vi "Rx Packet Page.vi"(8 "error in (no error)":errorcluster, 11 "Node Ptr":T2 format="%.0x") -> (0 "error out":errorcluster)   [LabVIEW 2023, in "UDP-Custom-Device System Explorer.lvlib"]
uses:
  UDP-Custom-Device System Explorer.lvlib
  Shared/Types/Shared - New Data Options.ctl
  <vilib>/NI VeriStand/Custom Device API/Custom Device Item Ref.ctl
  Types/Page References/Refs - Rx Packets Page.ctl
  Shared/Types/Shared - Channel Data Type.ctl
  <vilib>/NI VeriStand/Custom Device API/Custom Device API.lvlib
  Property Accessors/Shared Packet Accessors.lvlib
  <vilib>/NI VeriStand/Custom Device Tools/Custom Device Utility Library/Custom Device Utility Library.lvlib
  Property Accessors/Rx Channel Accessors.lvlib
  Property Accessors/Rx Packet Accessors.lvlib
  Property Accessors/Rx Channel Section Accessors.lvlib
  Shared/UDP-Custom-Device Shared.lvlib
panel:
  in  "Config Threading":bool
  in  "Debug Mode":bool caption="Auto-Assign Local NIC"
  in  "New Data Options":T1
  in  "Multicast IP Address":string
  in  "Multicast?":bool caption="Auto-Assign Local NIC"
  in  "Read Timeout (ms)":i32
  in  "Channel Config Export":bool
  in  "Configure Header":bool
  in  "Endianness":u16(ring) items=["big-endian"=0, "little-endian"=2]
  in  "General Header 3":cluster{"Section Name":string}={"Section Name"="Network Settings"}
  out "Packet ID":i32
  in  "Auto-Assign Local NIC":bool
  in  "Port":u16
  in  "IP Address of Local NIC":string
  in  "Description":string
  in  "Name":string
  in  "General Header 2":cluster{"Section Name":string}={"Section Name"="Configured Channels"}
  in  "Rx Channels":i32[](listbox)
  in  "SHDocVw.IWebBrowser":refnum<k7>(container)
  in  "General Header":cluster{"Section Name":string}={"Section Name"="Packet Configuration"}
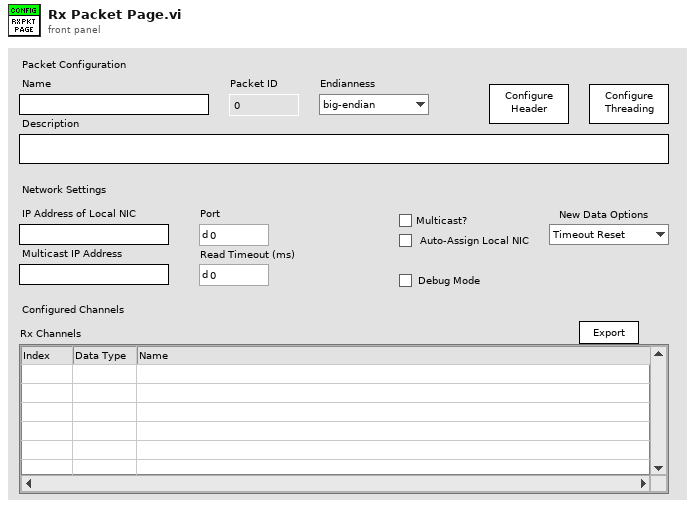
[diagram p1: front panel]
types:
  T1 = typedef "UDP-Custom-Device Shared.lvlib/Shared - New Data Options.ctl" = enum16{"Timeout Reset", "Counter"}
  T2 = typedef "Custom Device API.lvlib/Custom Device Item Ref.ctl" = u64
  T3 = typedef "UDP-Custom-Device System Explorer.lvlib/Refs - Rx Packets Page.ctl" = cluster{"Name":refnum<vi>, "Description":refnum<vi>, "Rx Packets":refnum<vi>, "Auto Assign Local NIC?":refnum<vi>, "IP Address of Local NIC":refnum<vi>, "Port":refnum<vi>, "Packet ID":refnum<vi>, "Channel Config Export":refnum<vi>, "Read Timeout (ms)":refnum<vi>, "Endianness":refnum<vi>, "Multicast IP Address":refnum<vi>, "Multicast?":refnum<vi>, "New Data Options":refnum<vi>, "Debug Mode":refnum<vi>}
  T4 = enum8{"Enabled", "Disabled", "Disabled and Grayed Out"}
  T5 = typedef "UDP-Custom-Device Shared.lvlib/Shared - Channel Data Type.ctl" = enum16{"Boolean", "Single", "Double", "I8", "I16", "I32", "I64", "U8", "U16", "U32", "U64"}
  T6 = typedef "Custom Device API.lvlib/Custom Device Commands.ctl" = enum16{"Default", "Item renamed", "Shutdown", "Dynamic button pressed"}
  T7 = typedef "UDP-Custom-Device System Explorer.lvlib/Thread Configuration.ctl" = cluster{"targetProcessor":i8, "targetPriority":i16, "Synchronization":T8, "loopPeriod":u32, "pclDecimation":u16, "threadManagement":T9}
  T8 = typedef "UDP-Custom-Device System Explorer.lvlib/Thread Sync Reference.ctl" = enum16{"PCL", "Async"}
  T9 = typedef "UDP-Custom-Device Shared.lvlib/Shared - Thread Management.ctl" = enum16{"Untimed (Default)", "Timed (High Priority)"}
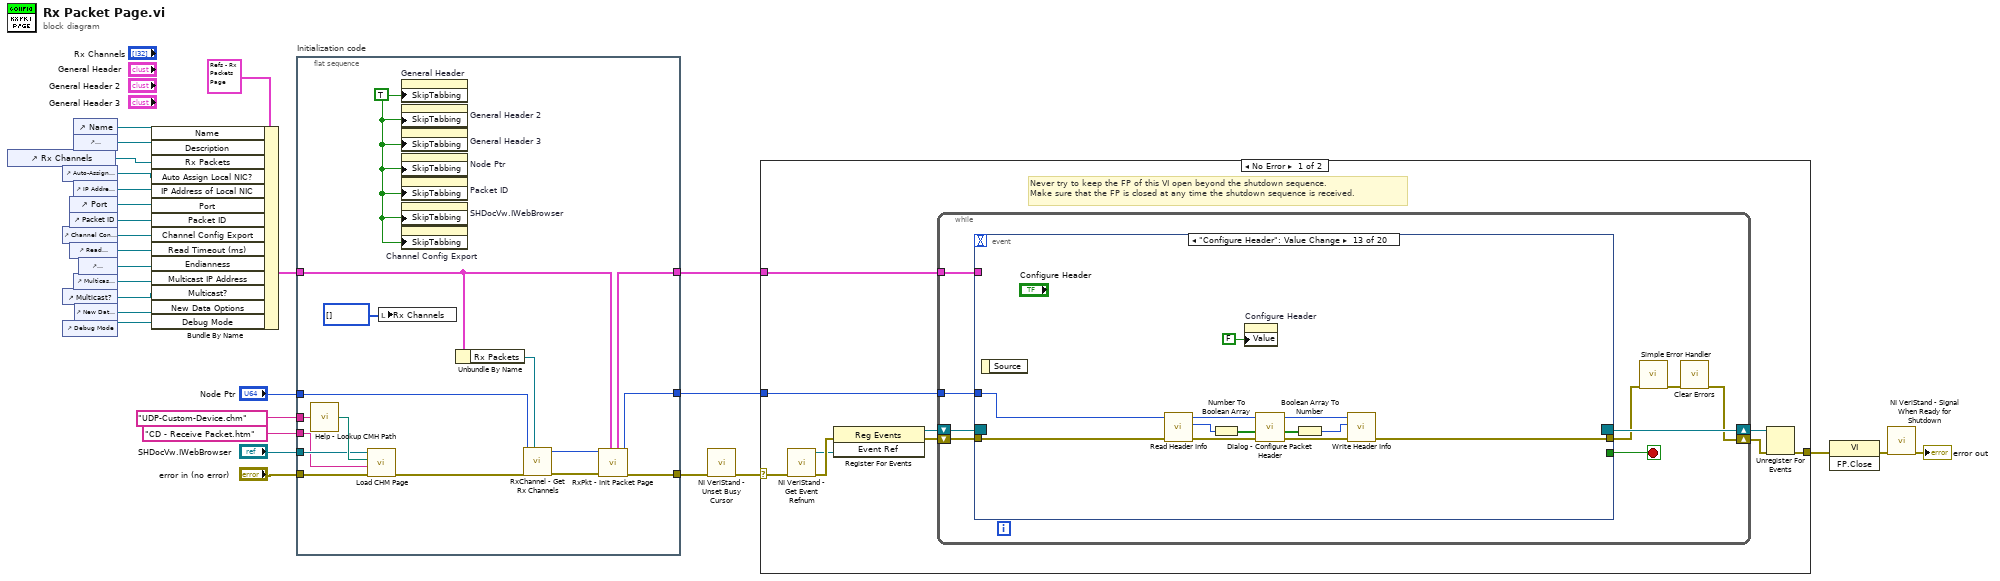
[diagram p0: block diagram]
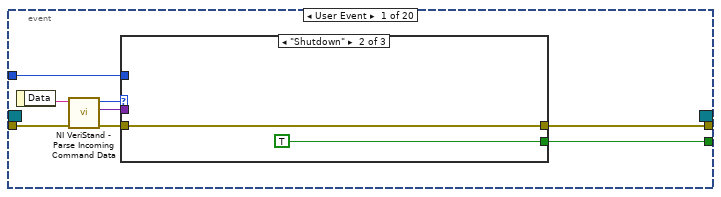
[diagram p2: hidden frame]
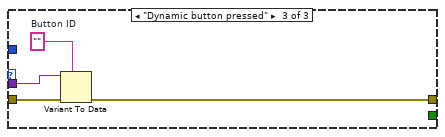
[diagram p4: hidden frame]
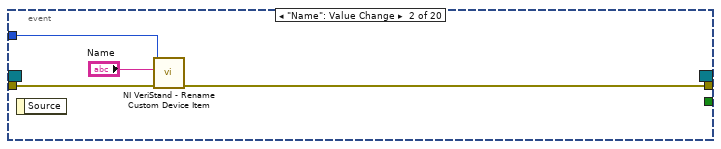
[diagram p5: hidden frame]
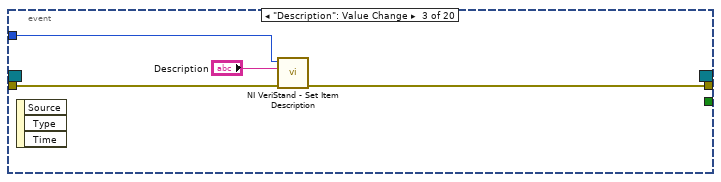
[diagram p6: hidden frame]
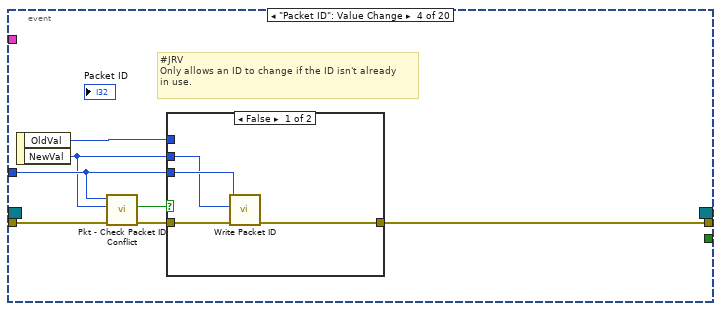
[diagram p7: hidden frame]
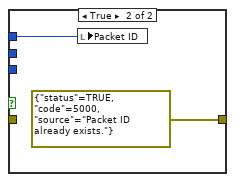
[diagram p8: hidden frame]
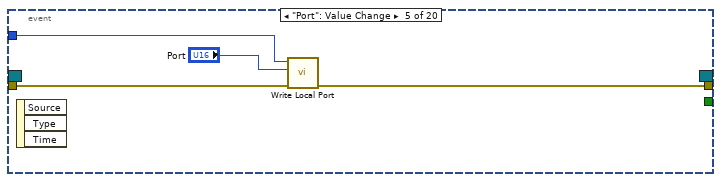
[diagram p9: hidden frame]
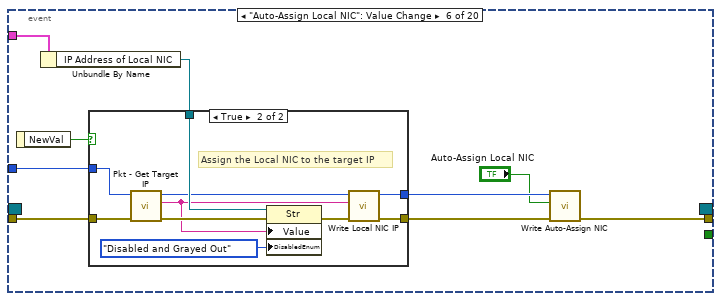
[diagram p10: hidden frame]
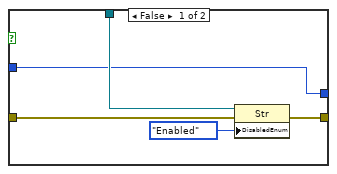
[diagram p11: hidden frame]
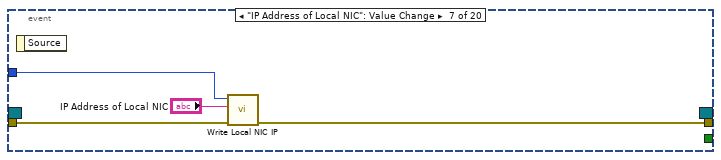
[diagram p12: hidden frame]
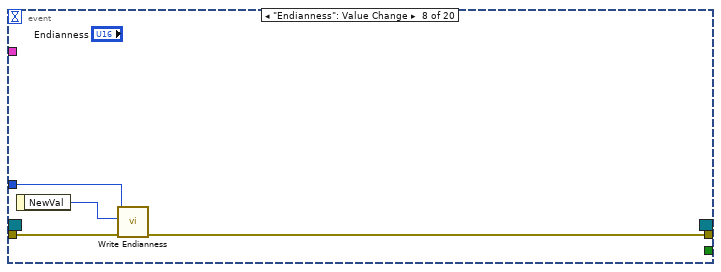
[diagram p13: hidden frame]
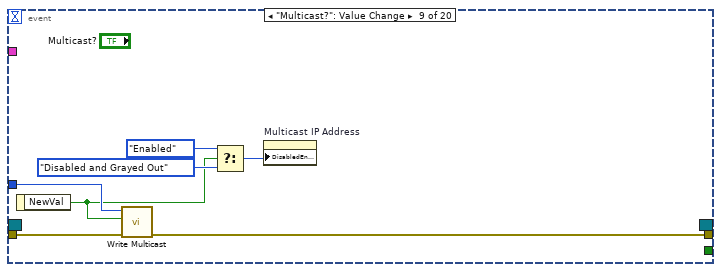
[diagram p14: hidden frame]
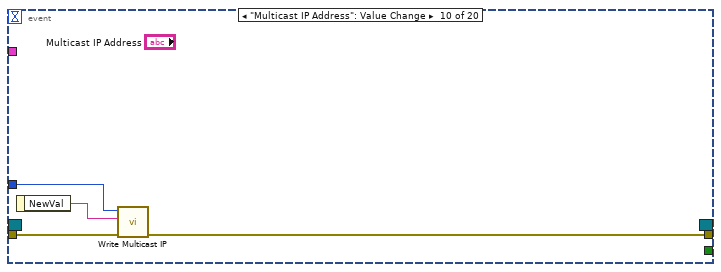
[diagram p15: hidden frame]
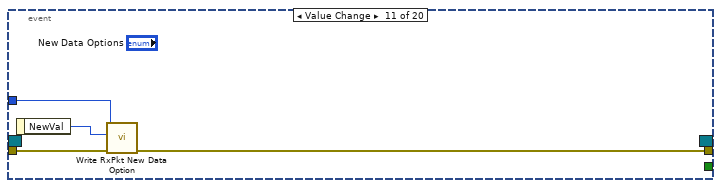
[diagram p16: hidden frame]
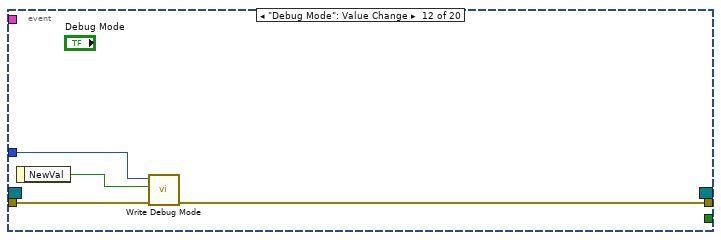
[diagram p17: hidden frame]
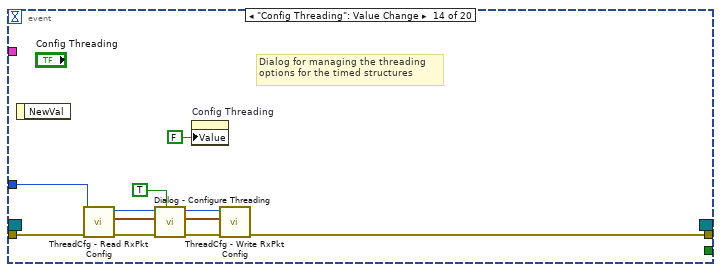
[diagram p18: hidden frame]
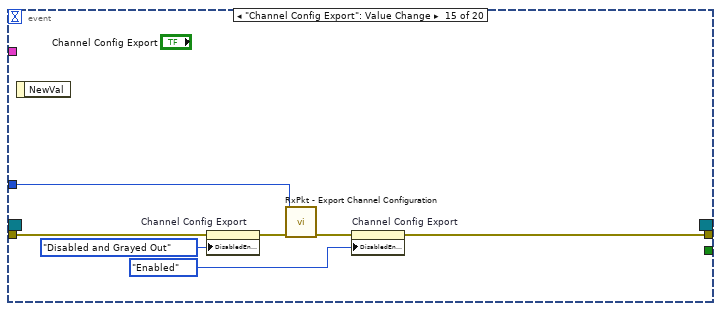
[diagram p19: hidden frame]
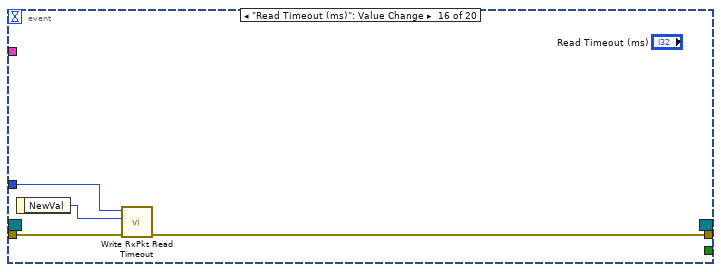
[diagram p20: hidden frame]
diagram:
  n1 = control-ref of="Rx Channels"() -> (w13:refnum<vi>)
  n2 = control-ref of="Auto-Assign Local NIC"() -> (w14:refnum<vi>)
  n3 = control-ref of="Channel Config Export"() -> (w7:refnum<vi>)
  n4 = control-ref of="Multicast?"() -> (w4:refnum<vi>)
  n5 = control-ref of="Debug Mode"() -> (w1:refnum<vi>)
  n6 = control-ref of="Port"() -> (w10:refnum<vi>)
  n7 = control-ref of="Packet ID"() -> (w12:refnum<vi>)
  n8 = control-ref of="Read Timeout (ms)"() -> (w6:refnum<vi>)
  n9 = control-ref of="Name"() -> (w16:refnum<vi>)
  n10 = control-ref of="Description"() -> (w15:refnum<vi>)
  n11 = control-ref of="IP Address of Local NIC"() -> (w11:refnum<vi>)
  n12 = control-ref of="Multicast IP Address"() -> (w3:refnum<vi>)
  n13 = control-ref of="New Data Options"() -> (w2:refnum<vi>)
  n14 = control-ref of="Endianness"() -> (w5:refnum<vi>)
  n15 = Bundle By Name(cluster=T3 {"Name"=refnum, "Description"=refnum, "Rx Packets"=refnum, "Auto Assign Local NIC?"=refnum, "IP Address of Local NIC"=refnum, "Port"=refnum, "Packet ID"=refnum, "Channel Config Export"=refnum, "Read Timeout (ms)"=refnum, "Endianness"=refnum, "Multicast IP Address"=refnum, "Multicast?"=refnum, "New Data Options"=refnum, "Debug Mode"=refnum} ("Rx Section Cluster"), "Name"=w16, "Description"=w15, "Rx Packets"=w13, "Auto Assign Local NIC?"=w14, "IP Address of Local NIC"=w11, "Port"=w10, "Packet ID"=w12, "Channel Config Export"=w7, "Read Timeout (ms)"=w6, "Endianness"=w5, "Multicast IP Address"=w3, "Multicast?"=w4, "New Data Options"=w2, "Debug Mode"=w1) -> (w9:T3)
  n16 = flat-sequence "Initialization code" {
    tunnel: "error in (no error)" -> [w38]
    tunnel: "Node Ptr" -> [w43]
    tunnel: [w31] -> w24
    tunnel: "SHDocVw.IWebBrowser" -> [w36]
    tunnel: "CD - Receive Packet.htm" ("CD_CHM_Section") -> [w35]
    tunnel: "UDP-Custom-Device.chm" ("CD_CHM_FileName") -> [w37]
    tunnel: w9 -> [w42]
    tunnel: [w41] -> w18
    tunnel: [w34] -> w8
    frame #0 {
      w29 = TRUE ("Skip When Tabbing")
      n17 = call "Help - Lookup CMH Path.vi"("Main CMH File"=w37) -> ("Compiled CMH Path"=w39:path)
      n18 = call <vilib>:"Load CHM Page.vi"("error in (no error)"=w38, "HTML File"=w35, "Compiled CHM Path"=w39, "Web Browser Reference"=w36) -> ("error out"=w30:errorcluster)  [unwired: 7 in]
      n19 = local write "Rx Channels"(i32[] [] ("Rx Channels")) -> ()
      n20 = property on="General Header" class="Clust (strict)"("SkipTabbing"=w29) -> ()  [unwired: 2 in, 2 out]
      n21 = property on="General Header 2" class="Clust (strict)"("SkipTabbing"=w29) -> ()  [unwired: 2 in, 2 out]
      n22 = property on="General Header 3" class="Clust (strict)"("SkipTabbing"=w29) -> ()  [unwired: 2 in, 2 out]
      n23 = property on="Node Ptr" class="DigNum (strict)"("SkipTabbing"=w29) -> ()  [unwired: 2 in, 2 out]
      n24 = property on="Packet ID" class="DigNum (strict)"("SkipTabbing"=w29) -> ()  [unwired: 2 in, 2 out]
      n25 = property on="SHDocVw.IWebBrowser" class="AXCont"("SkipTabbing"=w29) -> ()  [unwired: 2 in, 2 out]
      n26 = property on="Channel Config Export" class="Bool"("SkipTabbing"=w29) -> ()  [unwired: 2 in, 2 out]
      n27 = Unbundle By Name(w42) -> ("Rx Packets"=w44:refnum<vi>)
      n28 = call "RxChannel - Get Rx Channels.vi"("MCLB"=w44, "error in (no error)"=w30, "Node Ptr"=w43) -> ("error out"=w32:errorcluster, "Node Ptr out"=w40:T2)  [unwired: 6 in, 1 out]
      n29 = call "RxPkt - Init Packet Page.vi"("Rx Section Cluster In"=w42, "error in (no error)"=w32, "Node Ptr In"=w40) -> ("error out"=w31:errorcluster, "Node Ptr Out"=w34:T2, "Rx Section Cluster Out"=w41:T3)  [unwired: 6 in]
    }
  }
  n30 = call <vilib>:"NI VeriStand - Unset Busy Cursor.vi"("error in (no error)"=w24) -> ("error out"=w23:errorcluster)  [unwired: 10 out]
  n31 = case shown="No Error" w23 {
    selector: w23 -> [w46 w270]
    tunnel: [w51 w268] -> w28
    tunnel: w8 -> [w47 _]
    tunnel: w18 -> [w45 _]
    frame No Error {
      # "Never try to keep the FP of this VI open beyond the shutdown sequence.\nMake sure that the FP is closed at any time the shutdown sequence is received."
      n32 = call <vilib>:"NI VeriStand - Get Event Refnum.vi"("error in (no error)"=w46) -> ("error out"=w54:errorcluster, "Event Ref"=w50:refnum<user-event>)  [unwired: 9 out]
      n33 = register-events(error in=w54, w50) -> (reference out=w48:refnum<event-registration>, error out=w49:errorcluster)  [unwired: 1 in]
      n34 = while {
        tunnel: w47 -> [w59]
        shift-right: [w56] -> w52
        shift-left: w49 -> [w62]
        shift-right: [w63] -> w53
        shift-left: w48 -> [w61]
        tunnel: w45 -> [w55]
        stop <- w60 stop-if-true
        n35 = event shown="[12] \"Configure Header\": Value Change" {
          selector: w61 -> [_ _ _ _ _ _ _ _ _ _ _ _ _ _ _ _ _ _ _ _]
          dyn-events: [_ _ _ _ _ _ _ _ _ _ _ _ _ _ _ _ _ _ _ _] -> w63
          timeout: _ -> [_ _ _ _ _ _ _ _ _ _ _ _ _ _ _ _ _ _ _ _]
          tunnel: w62 -> [w71 w82 w86 w91 w102 w112 w131 w134 w141 w144 w148 w153 w163 w176 w183 w188 w190 w203 _ w225]
          tunnel: [w67 _ _ _ _ _ _ _ _ _ _ _ _ _ _ _ _ _ _ _] -> w60
          tunnel: [w66 w80 w83 w93 w101 w105 w130 w133 w140 w143 w147 w151 w157 w170 w180 w185 w189 w200 _ w226] -> w58
          tunnel: w59 -> [w65 w81 w85 w92 w103 w111 w128 w135 w142 w146 w150 w154 w164 w175 w184 w187 w191 w204 _ w224]
          tunnel: w55 -> [_ _ _ _ _ w108 _ _ _ _ _ _ _ _ _ _ _ _ _ _]
          event User Event {
            n36 = event-data() -> ("Data"=w70:string)  [unwired: 1 out]
            n37 = call <vilib>:"NI VeriStand - Parse Incoming Command Data.vi"("error in (no error)"=w71, "Incoming data"=w70) -> ("error out"=w69:errorcluster, "Outgoing data"=w64:variant, "Action"=w68:T6)  [unwired: 7 out]
            n38 = case shown="\"Shutdown\"" w68 {
              tunnel: w69 -> [w72 w73 w78]
              tunnel: [_ TRUE _] -> w67
              tunnel: [w72 w73 w75] -> w66
              tunnel: w65 -> [_ _ _]
              tunnel: w64 -> [_ _ w77]
              frame "Default", Default {
              }
              frame "Shutdown" {
              }
              frame "Dynamic button pressed" {
                w76 = ""  # Button ID
                n39 = Variant To Data(error in=w78, type=w76, Variant=w77) -> (error out=w75:errorcluster)  [unwired: 1 out]
              }
            }
          }
          event "Name": Value Change {
            n40 = event-data() -> ()  [unwired: 2 out]
            n41 = call <vilib>:"NI VeriStand - Rename Custom Device Item.vi"("error in (no error)"=w82, "New Name"="Name", "Item Ref in"=w81) -> ("error out"=w80:errorcluster)  [unwired: 6 in, 2 out]
          }
          event "Description": Value Change {
            n42 = event-data() -> ()  [unwired: 4 out]
            n43 = call <vilib>:"NI VeriStand - Set Item Description.vi"("error in (no error)"=w86, "Description"="Description", "Item Ref in"=w85) -> ("error out"=w83:errorcluster)  [unwired: 6 in, 2 out]
          }
          event "Packet ID": Value Change {
            # "#JRV\nOnly allows an ID to change if the ID isn't already\nin use."
            n44 = event-data() -> ("OldVal"=w87:i32, "NewVal"=w88:i32)  [unwired: 1 out]
            n45 = call "Pkt - Check Packet ID Conflict.vi"("error in (no error)"=w91, "New ID"=w88, "Packet Ref In"=w92) -> ("error out"=w90:errorcluster, "Conflicting ID?"=w89:bool)  [unwired: 7 in]
            n46 = case shown="False" w89 {
              tunnel: [w96 errorcluster {"status"=TRUE, "code"=5000, "source"="Packet ID already exists."} ("error out")] -> w93
              tunnel: w92 -> [w95 _]
              tunnel: w90 -> [w97 _]
              tunnel: w88 -> [w94 _]
              tunnel: w87 -> [_ w99]
              frame False {
                n47 = call "Write Packet ID.vi"("error in (no error)"=w97, "Packet ID"=w94, "Node Ptr"=w95) -> ("error out"=w96:errorcluster)  [unwired: 7 in, 1 out]
              }
              frame True {
                n48 = local write "Packet ID"(w99) -> ()
              }
            }
          }
          event "Port": Value Change {
            n49 = event-data() -> ()  [unwired: 4 out]
            n50 = call "Write Local Port.vi"("error in (no error)"=w102, "Port"="Port", "Node Ptr"=w103) -> ("error out"=w101:errorcluster)  [unwired: 7 in, 1 out]
          }
          event "Auto-Assign Local NIC": Value Change {
            n51 = event-data() -> ("NewVal"=w110:bool)  [unwired: 1 out]
            n52 = Unbundle By Name(w108) -> ("IP Address of Local NIC"=w109:refnum<vi>)
            n53 = case shown="True" w110 {
              tunnel: w111 -> [w114 w126]
              tunnel: w109 -> [w115 w124]
              tunnel: w112 -> [w116 w127]
              tunnel: [w117 w118] -> w106
              tunnel: [w114 w121] -> w107
              frame False {
                n54 = property class="Str"(reference=w115, error in=w116, "DisabledEnum"=T4."Enabled" ("Disabled")) -> (error out=w117:errorcluster)  [unwired: 1 out]
              }
              frame True {
                # "Assign the Local NIC to the target IP"
                n55 = call "Pkt - Get Target IP.vi"("error in"=w127, "Item Ref in"=w126) -> ("error out"=w125:errorcluster, "IPAddress"=w120:string, "Item Ref out"=w122:T2)  [unwired: 7 in]
                n56 = property class="Str"(reference=w124, error in=w125, "Value"=w120, "DisabledEnum"=T4."Disabled and Grayed Out" ("Disabled")) -> (error out=w119:errorcluster)  [unwired: 1 out]
                n57 = call "Write Local NIC IP.vi"("error in (no error)"=w119, "IP Address of Local NIC"=w120, "Node Ptr"=w122) -> ("error out"=w118:errorcluster, "Node Ptr out"=w121:T2)  [unwired: 7 in]
              }
            }
            n58 = call "Write Auto-Assign NIC.vi"("error in (no error)"=w106, "Auto-Assign NIC"="Auto-Assign Local NIC", "Node Ptr"=w107) -> ("error out"=w105:errorcluster)  [unwired: 7 in, 1 out]
          }
          event "IP Address of Local NIC": Value Change {
            n59 = event-data() -> ()  [unwired: 2 out]
            n60 = call "Write Local NIC IP.vi"("error in (no error)"=w131, "IP Address of Local NIC"="IP Address of Local NIC", "Node Ptr"=w128) -> ("error out"=w130:errorcluster)  [unwired: 7 in, 1 out]
          }
          event "Endianness": Value Change {
            n61 = event-data() -> ("NewVal"=w132:u16)  [unwired: 1 out]
            n62 = call "Write Endianness.vi"("error in (no error)"=w134, "Endianness"=w132, "Node Ptr"=w135) -> ("error out"=w133:errorcluster)  [unwired: 7 in, 1 out]
          }
          event "Multicast?": Value Change {
            n63 = event-data() -> ("NewVal"=w137:bool)  [unwired: 1 out]
            n64 = call "Write Multicast.vi"("error in (no error)"=w141, "Multicast"=w137, "Node Ptr"=w142) -> ("error out"=w140:errorcluster)  [unwired: 7 in, 1 out]
            n65 = Select(t=T4."Enabled" ("Disabled"), s=w137, f=T4."Disabled and Grayed Out" ("Disabled")) -> (s? t:f=w136:T4)
            n66 = property on="Multicast IP Address" class="Str"("DisabledEnum"=w136) -> ()  [unwired: 2 in, 2 out]
          }
          event "Multicast IP Address": Value Change {
            n67 = event-data() -> ("NewVal"=w145:string)  [unwired: 1 out]
            n68 = call "Write Multicast IP.vi"("error in (no error)"=w144, "Multicast IP Address"=w145, "Node Ptr"=w146) -> ("error out"=w143:errorcluster)  [unwired: 7 in, 1 out]
          }
          event Value Change {
            n69 = event-data() -> ("NewVal"=w149:T1)  [unwired: 1 out]
            n70 = call "Write RxPkt New Data Option.vi"("error in (no error)"=w148, "New Data Option"=w149, "Node Ptr"=w150) -> ("error out"=w147:errorcluster)  [unwired: 7 in, 1 out]
          }
          event "Debug Mode": Value Change {
            n71 = event-data() -> ("NewVal"=w152:bool)  [unwired: 1 out]
            n72 = call "Write Debug Mode.vi"("error in (no error)"=w153, "Debug Mode"=w152, "Node Ptr"=w154) -> ("error out"=w151:errorcluster)  [unwired: 7 in, 1 out]
          }
          event "Configure Header": Value Change {
            n73 = event-data() -> ()  [unwired: 2 out]
            n74 = call "Read Header Info.vi"("error in (no error)"=w163, "Node Ptr"=w164) -> ("error out"=w162:errorcluster, "Header Info"=w161:u32, "Node Ptr out"=w160:T2)  [unwired: 7 in]
            n75 = Number To Boolean Array(number=w161) -> (Boolean array=w166:bool[])
            n76 = property on="Configure Header" class="Bool (strict)"("Value"=FALSE ("Configure Header")) -> ()  [unwired: 2 in, 2 out]
            n77 = call "Dialog - Configure Packet Header.vi"("error in (no error)"=w162, "Header Elements In"=w166, "Packet Ref in"=w160) -> ("error out"=w158:errorcluster, "Header Elements Out"=w165:bool[], "Packet Ref out"=w159:T2)  [unwired: 6 in]
            n78 = Boolean Array To Number(Boolean array=w165) -> (number=w156:u32)
            n79 = call "Write Header Info.vi"("error in (no error)"=w158, "Header Info"=w156, "Node Ptr"=w159) -> ("error out"=w157:errorcluster)  [unwired: 7 in, 1 out]
          }
          event "Config Threading": Value Change {
            # "Dialog for managing the threading\noptions for the timed structures"
            n80 = event-data() -> ()  [unwired: 2 out]
            n81 = call "ThreadCfg - Read RxPkt Config.vi"("error in (no error)"=w176, "Node Ptr In"=w175) -> ("error out"=w169:errorcluster, "threadOptions"=w174:T7, "Node Ptr Out"=w168:T2)  [unwired: 7 in]
            n82 = call "Dialog - Configure Threading.vi"("rxPacket?"=TRUE, "error in (no error)"=w169, "threadOptions in"=w174, "Packet Ref in"=w168) -> ("error out"=w172:errorcluster, "threadOptions out"=w171:T7, "Packet Ref out"=w173:T2)  [unwired: 4 in]
            n83 = property on="Config Threading" class="Bool (strict)"("Value"=FALSE ("Config Threading")) -> ()  [unwired: 2 in, 2 out]
            n84 = call "ThreadCfg - Write RxPkt Config.vi"("error in (no error)"=w172, "threadOptions"=w171, "Node Ptr In"=w173) -> ("error out"=w170:errorcluster)  [unwired: 7 in, 1 out]
          }
          event "Channel Config Export": Value Change {
            n85 = event-data() -> ()  [unwired: 2 out]
            n86 = property on="Channel Config Export" class="Bool"(error in=w183, "DisabledEnum"=T4."Disabled and Grayed Out" ("Disabled")) -> (error out=w182:errorcluster)  [unwired: 1 in, 1 out]
            n87 = call "RxPkt - Export Channel Configuration.vi"("error in (no error)"=w182, "Packet Ref in"=w184) -> ("error out"=w181:errorcluster)  [unwired: 8 in, 1 out]
            n88 = property on="Channel Config Export" class="Bool"(error in=w181, "DisabledEnum"=T4."Enabled" ("Disabled")) -> (error out=w180:errorcluster)  [unwired: 1 in, 1 out]
          }
          event "Read Timeout (ms)": Value Change {
            n89 = event-data() -> ("NewVal"=w186:i32)  [unwired: 1 out]
            n90 = call "Write RxPkt Read Timeout.vi"("error in (no error)"=w188, "Read Timeout"=w186, "Node Ptr"=w187) -> ("error out"=w185:errorcluster)  [unwired: 7 in, 1 out]
          }
          event "Rx Channels": Value Change {
            n91 = event-data() -> ()  [unwired: 2 out]
            n92 = property on="Rx Channels" class="MCListbox (strict)"() -> ("ItemNames"=w193:string[][], "Value"=w194:i32[])  [unwired: 2 in, 2 out]
            n93 = for {
              tunnel: w193 -> [w198]
              tunnel: [w197] -> w192 mode=indexing
              tunnel: w194 -> [w196] mode=indexing
              n94 = Index Array(array=w198, index (row)=w196, index (col)=2 ("disabled index (row)")) -> (element=w197:string)
            }
            n95 = call "Write Selected Channels.vi"("error in (no error)"=w190, "Selected Channel Names"=w192, "Node Ptr"=w191) -> ("error out"=w189:errorcluster)  [unwired: 7 in, 1 out]
          }
          event "Rx Channels": Drag Ended {
            n96 = event-data() -> ("CtlRef"=w213:refnum<vi>)  [unwired: 1 out]
            n97 = property class="MCListbox (strict)"(reference=w213) -> ("ItemNames"=w205:string[][])  [unwired: 1 in, 2 out]
            n98 = Index Array(array=w205, index (col)=0 ("disabled index (col)")) -> (element=w208:string[])  [unwired: 1 in]
            n99 = Index Array(array=w205, index (col)=2 ("index (row)")) -> (element=w199:string[])  [unwired: 1 in]
            n100 = Array Size(array=w208) -> (size(s)=w209:i32)
            n101 = call "Write Selected Channels.vi"("error in (no error)"=w203, "Selected Channel Names"=w199, "Node Ptr"=w204) -> ("error out"=w201:errorcluster, "Node Ptr out"=w202:T2)  [unwired: 7 in]
            n102 = for {
              N: w209 -> [_]
              tunnel: [w214] -> w211 mode=indexing
              i -> [w216]
              n103 = Number To Decimal String(number=w216, width (-)=i16 3) -> (decimal integer string=w214:string)
            }
            n104 = call "RxChannel - Update Rx Channel Order.vi"("Channel Names"=w199, "error in (no error)"=w201, "Node Ptr"=w202) -> ("error out"=w200:errorcluster)  [unwired: 7 in, 1 out]
            n105 = Replace Array Subset(array=w205, new element=w211, index (col)=0 ("disabled index (col)")) -> (w206:string[][])  [unwired: 1 in]
            n106 = property class="MCListbox (strict)"(reference=w213, "ItemNames"=w206) -> ()  [unwired: 1 in, 2 out]
          }
          event "Rx Channels": Shortcut Menu Activation? {
            n107 = event-data() -> ("MenuRef"=w223:refnum<k9>)  [unwired: 1 out]
            n108 = Insert Menu Items(7:string[] ["RemoveChannels", "ChangeType"] ("item names"), 8:string[] ["Remove Channels", "Change Type"] ("item names"), 9:w223) -> (3:w220:refnum<k9>)  [unwired: 3 in, 2 out]
            n109 = call "Pkt - Menu Data Types.vi"() -> ("Menu Tags"=w217:string[], "Menu Names"=w218:string[])  [unwired: 10 in]
            n110 = Insert Menu Items(5:"ChangeType", 7:w217, 8:w218, 9:w220) -> ()  [unwired: 2 in, 3 out]
            n111 = event-data() -> ()  [unwired: 2 in, 1 out]
          }
          event "Rx Channels": Shortcut Menu Selection (User) {
            n112 = event-data() -> ("ItemTag"=w227:string)  [unwired: 1 out]
            n113 = case shown="\"RemoveChannels\"" w227 {
              selector: w227 -> [_ w242]
              tunnel: [w228 w245] -> w226
              tunnel: w225 -> [w234 w251]
              tunnel: w224 -> [w230 w243]
              frame "RemoveChannels" {
                n114 = call "RxChannel - Remove Rx Channels.vi"("error in (no error)"=w234, "Node Ptr"=w230) -> ("error out"=w229:errorcluster)  [unwired: 9 in]
                n115 = property on="Rx Channels" class="MCListbox (strict)"() -> ("ItemNames"=w233:string[][], "Value"=w231:i32[])  [unwired: 2 in, 2 out]
                n116 = for {
                  tunnel: w231 -> [w239]
                  tunnel: [w240] -> w232 mode=indexing if=w236
                  tunnel: w233 -> [w240] mode=indexing
                  i -> [w238]
                  n117 = Search 1D Array(1D array=w239, element=w238) -> (index of element=w237:i32)  [unwired: 1 in]
                  n118 = Less Than 0?(x=w237) -> (x < 0?=w236:bool)
                }
                n119 = call <vilib>:"NI VeriStand - Highlight Node in System Explorer.vi"("error in (no error)"=w229, "Item Ref in"=w230) -> ("error out"=w228:errorcluster)  [unwired: 8 in, 1 out]
                n120 = property on="Rx Channels" class="MCListbox (strict)"("ItemNames"=w232, "Value"=i32[] [] ("Rx Channels")) -> ()  [unwired: 2 in, 2 out]
              }
              frame Default {
                n121 = case shown="\"CTBoolean\"" w242 {
                  tunnel: [Shared_-_Channel_Data_Type."Single" ("Data Type") Shared_-_Channel_Data_Type."Double" ("Data Type") Shared_-_Channel_Data_Type."Boolean" ("Data Type") Shared_-_Channel_Data_Type."I8" ("Data Type") Shared_-_Channel_Data_Type."I16" ("Data Type") Shared_-_Channel_Data_Type."I32" ("Data Type") Shared_-_Channel_Data_Type."I64" ("Data Type") Shared_-_Channel_Data_Type."U8" ("Data Type") Shared_-_Channel_Data_Type."U16" ("Data Type") Shared_-_Channel_Data_Type."U32" ("Data Type") Shared_-_Channel_Data_Type."U64" ("Data Type")] -> w241
                  frame "CTSingle", Default {
                  }
                  frame "CTDouble" {
                  }
                  frame "CTBoolean" {
                  }
                  frame "CTI8" {
                  }
                  frame "CTI16" {
                  }
                  frame "CTI32" {
                  }
                  frame "CTI64" {
                  }
                  frame "CTU8" {
                  }
                  frame "CTU16" {
                  }
                  frame "CTU32" {
                  }
                  frame "CTU64" {
                  }
                }
                n122 = local read "Rx Channels"() -> (w247:i32[])
                n123 = call <vilib>:"NI VeriStand - Get Item Reference by Name.vi"("error in (no error)"=w251, "Item Name"="Channels" ("Section Name"), "Parent Ref in"=w243) -> ("error out"=w248:errorcluster, "Item Ref"=w249:T2)  [unwired: 5 in, 2 out]
                n124 = call "Read Rx Channel Dependent Nodes.vi"("error in (no error)"=w248, "Node Ptr"=w249) -> ("Dependent Node Refs"=w246:T2[])  [unwired: 7 in, 2 out]
                n125 = for {
                  tunnel: w247 -> [w266] mode=indexing
                  tunnel: w246 -> [w267]
                  tunnel: w241 -> [w264]
                  tunnel: [w263] -> w244
                  n126 = Index Array(array=w267, index=w266) -> (element=w265:T2)
                  n127 = call "Write Rx Data Type.vi"("Data Type"=w264, "Node Ptr"=w265) -> ("error out"=w263:errorcluster)  [unwired: 8 in, 1 out]
                }
                n128 = call <vilib>:"NI VeriStand - Highlight Node in System Explorer.vi"("error in (no error)"=w244, "Item Ref in"=w243) -> ("error out"=w245:errorcluster)  [unwired: 8 in, 1 out]
              }
            }
          }
        }
        n129 = call <vilib>:"Simple Error Handler.vi"("error in (no error)"=w58) -> ("error out"=w57:errorcluster)  [unwired: 1 in, 7 out]
        n130 = call <vilib>:"Clear Errors.vi"("error in (no error)"=w57) -> ("error out"=w56:errorcluster)  [unwired: 1 in, 5 out]
      }
      n131 = Unregister For Events(event registration refnum=w53, error in=w52) -> (error out=w51:errorcluster)
    }
    frame Error {
      n132 = call <vilib>:"Simple Error Handler.vi"("error in (no error)"=w270) -> ("error out"=w269:errorcluster)  [unwired: 1 in, 7 out]
      n133 = call <vilib>:"Clear Errors.vi"("error in (no error)"=w269) -> ("error out"=w268:errorcluster)  [unwired: 1 in, 5 out]
    }
  }
  n134 = invoke class="VI" method="FP.Close"(error in=w28) -> (error out=w27:errorcluster)  [unwired: 2 in, 2 out]
  n135 = call <vilib>:"NI VeriStand - Signal When Ready for Shutdown.vi"("error in (no error)"=w27) -> ("error out"=→"error out":errorcluster)  [unwired: 10 out]
